vi "Func_AddDataType.vi"(6 "Library Path":path, 8 "error in (no error)":errorcluster, 10 "Control Path":path=path "C:/Users/dsmith.AMER/Desktop/Control 1.ctl", 11 "data type name":string) -> (0 "error out":errorcluster, 4 "Polymorph count":i32)   [LabVIEW 2010, in "TemplateGenerator.lvlib"]
uses:
  TemplateGenerator.lvlib
  Type Defs/Data Types.ctl
  Current Value Table.lvlib
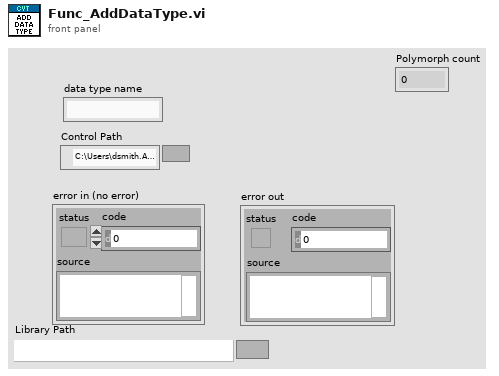
[diagram p1: front panel]
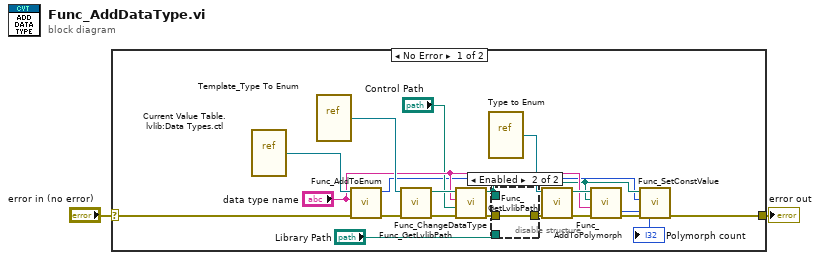
[diagram p0: block diagram]
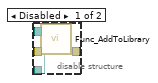
[diagram p2: hidden frame]
diagram:
  n1 = case shown="No Error" "error in (no error)" {
    selector: "error in (no error)" -> [w20 w27]
    tunnel: [w6 w27] -> w2
    frame No Error {
      n2 = vi-ref "Current Value Table.lvlib:Data Types.ctl"() -> (w21:refnum<vi>)
      n3 = vi-ref "Template_Type To Enum.vi"() -> (w16:refnum<vi>)
      n4 = call "Func_AddToEnum.vi"("error in (no error)"=w20, "data type name"="data type name", "VI in"=w21) -> ("error out"=w19:errorcluster, "NumItems"=w7:u32)  [unwired: 7 in]
      n5 = call "Func_GetLvlibPath.vi"("error in (no error)"=w19, "VI in"=w16) -> ("error out"=w13:errorcluster, "VI Path"=w15:path)  [unwired: 8 in]
      n6 = call "Func_ChangeDataType.vi"("error in (no error)"=w13, "Control Path"="Control Path", "data type name"="data type name", "template"=w15) -> ("error out"=w11:errorcluster, "Final Path"=w8:path)  [unwired: 6 in]
      n7 = vi-ref "Type to Enum.vi"() -> (w5:refnum<vi>)
      n8 = disable-structure shown="Enabled" {
        disable-tunnel: w11 -> [w25 w26]
        disable-tunnel: [w24 w26] -> w10
        disable-tunnel: w8 -> [w23 _]
        disable-tunnel: "Library Path" -> [w22 _]
        frame Disabled {
          n9 = call "Func_AddToLibrary.vi"("error in (no error)"=w25, "Library Path"=w22, "VI Path"=w23) -> ("error out"=w24:errorcluster)  [unwired: 8 in]
        }
        frame Enabled {
        }
      }
      n10 = call "Func_GetLvlibPath.vi"("error in (no error)"=w10, "VI in"=w5) -> ("error out"=w17:errorcluster, "VI Path"=w18:path)  [unwired: 8 in]
      n11 = call "Func_AddToPolymorph.vi"("error in (no error)"=w17, "Name"="data type name", "New VI's Path"=w8, "Polymorphic VI Path"=w18) -> ("error out"=w9:errorcluster, "Polymorph count"=→"Polymorph count":i32)  [unwired: 6 in]
      n12 = call "Func_SetConstValue.vi"("error in (no error)"=w9, "Number of Items"=w7, "VI's Path"=w8) -> ("error out"=w6:errorcluster)  [unwired: 8 in]
    }
    frame Error {
    }
  }
  "error out" <- w2
